vi "SetIOPinPulWidth.vi"(8 "错误输入（无错误）":errorcluster, 9 "SelPinType":i32, 10 "脉冲宽度值":u16, 11 "SelPinNum":i32) -> (0 "错误输出":errorcluster)   [LabVIEW 2014]
uses:
  X86Dll/ZXUTConfigMgr.dll
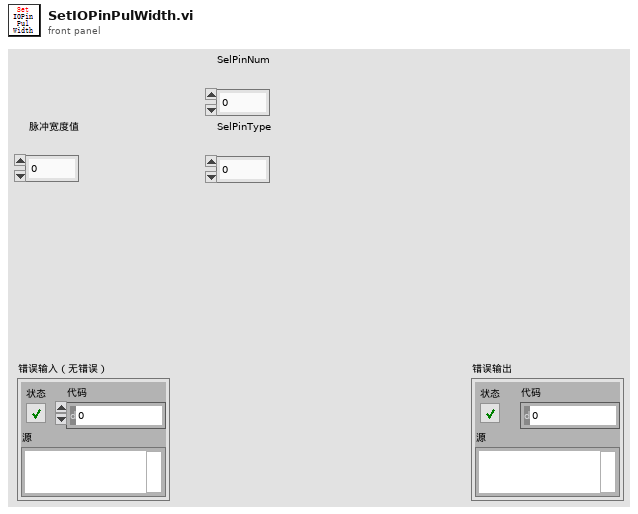
[diagram p1: front panel]
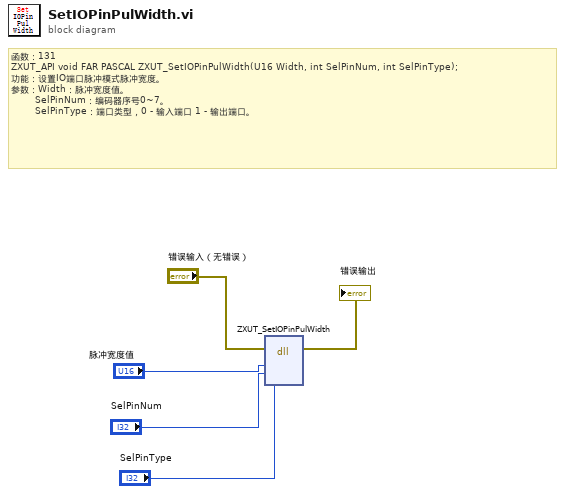
[diagram p0: block diagram]
diagram:
  # "函数：131\nZXUT_API void\tFAR PASCAL ZXUT_SetIOPinPulWidth(U16 Width, int SelPinNum, int SelPinType);\n功能：设置IO端口脉冲模式脉冲宽度。\n参数：Width：脉冲宽度值。\n        SelPinNum：编码器序号0~7。\n        SelPinType：端口类型，0 - 输入端口 1 - 输出端口。"
  n1 = dll-call lib="D:/Software/Utrasonic on-line monitoring/X86Dll/ZXUTConfigMgr.dll" fn="ZXUT_SetIOPinPulWidth"(error in="错误输入（无错误）", "Width"="脉冲宽度值", "SelPinNum"="SelPinNum", "SelPinType"="SelPinType") -> (error out=→"错误输出":errorcluster)  [unwired: 6 in, 1 out]
